vi "ze internal closure miss check.vi"(8 "error in (no error)":errorcluster, 11 "this_":cluster{"_context":u64, "_call":u64}) -> (0 "error out":errorcluster, 3 "function return":bool)   [LabVIEW 2021, in "zenohc.lvlib"]
doc: "bool ze_internal_closure_miss_check(const struct ze_owned_closure_miss_t *this_);"
uses:
  zenohc.lvlib
  zenohc.dll
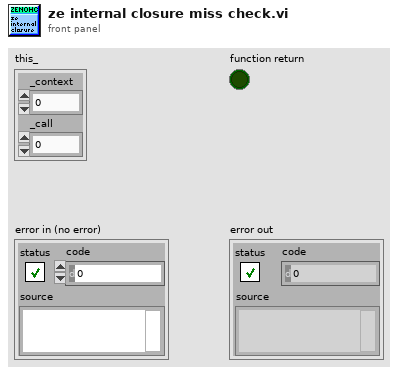
[diagram p1: front panel]
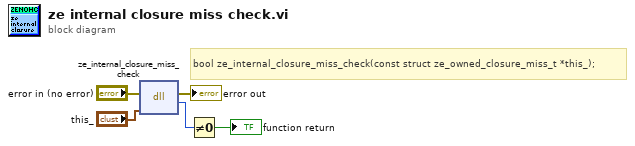
[diagram p0: block diagram]
diagram:
  # "bool ze_internal_closure_miss_check(const struct ze_owned_closure_miss_t *this_);"
  n1 = dll-call lib="D:/dev/zenoh_labview/zenohc/zenohc.*" fn="ze_internal_closure_miss_check"(error in="error in (no error)", "this_"="this_") -> (error out=→"error out":errorcluster, w4:u8)  [unwired: 3 in, 1 out]
  n2 = Not Equal To 0?(x=w4) -> (x != 0?=→"function return":bool)
